vi "Sync Config from Instr.vi"(8 "error in (no error)":errorcluster, 11 "LakeShore 336 Driver in":refnum<class "LakeShore 336 Driver.lvclass">) -> (0 "error out":errorcluster, 2 "Variant":variant, 3 "LakeShore 336 Driver out":refnum<class "LakeShore 336 Driver.lvclass">)   [LabVIEW 2024, in "LakeShore 336 Driver.lvclass"]
uses:
  LakeShore 336 Driver.lvclass
  D:/GitHub/NHMFL_Core/Libraries/Instruments/VISA Instrument/VISA Instrument.lvclass
  D:/GitHub/NHMFL_Core/Libraries/Instruments/Temperature Controller Driver/Temperature Controller Driver.lvclass
  VISA Instrument/VISA Instrument.lvclass/VISA Instrument.ctl
  VISA Instrument/Read VISA resource.vi
  VISA Instrument/Write VISA resource.vi
  Temperature Controller Driver/Read T controller configuration.vi
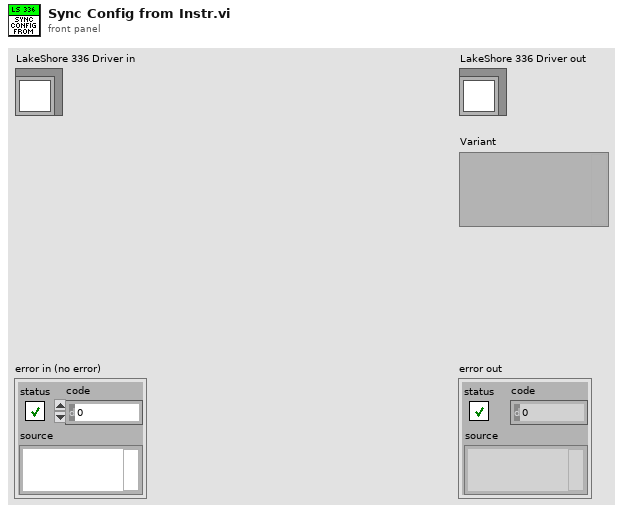
[diagram p1: front panel]
types:
  T1 = typedef "T controller configuration.ctl" = cluster{"Record Channels":string[], "Record raw signal":bool, "Set point":dbl, "Record heater":bool, "Ramp rate":dbl, "P":dbl, "I":dbl, "D":dbl, "Control":T2, "P manual":dbl, "Output #":i32}
  T2 = typedef "Control Mode.ctl" = enum16{"Off", "PID", "Ramp", "Manual", "Table"}
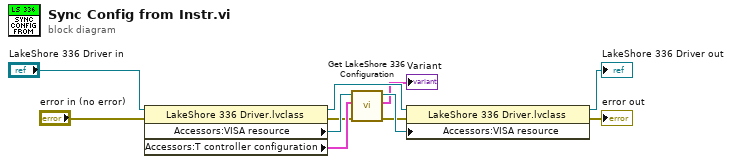
[diagram p0: block diagram]
diagram:
  n1 = property class="LakeShore 336 Driver.lvclass"(reference="LakeShore 336 Driver in", error in="error in (no error)") -> (reference out=w11:refnum<class "LakeShore 336 Driver.lvclass">, error out=w7:errorcluster, "Accessors:VISA resource"=w10:refnum<visa-resource-name>, "Accessors:T controller configuration"=w9:T1)
  n2 = call "Get LakeShore 336 Configuration.vi"("error in (no error)"=w7, "Config in"=w9, "VISA Resource Name"=w10) -> ("error out"=w6:errorcluster, "Config out"=→"Variant":T1, "VISA Resource Name Out"=w8:refnum<visa-resource-name>)  [unwired: 6 in]
  n3 = property class="LakeShore 336 Driver.lvclass"(reference=w11, error in=w6, "Accessors:VISA resource"=w8) -> (reference out=→"LakeShore 336 Driver out":refnum<class "LakeShore 336 Driver.lvclass">, error out=→"error out":errorcluster)
